vi "Remove Unnecessary Whitespace from XML.vi"(1 "Input":string) -> (0 "Output":string)   [LabVIEW 2018, in "VILab.lvlib"]
doc: "For easier comparison with generated XML to diagnose issues."
uses:
  VILab.lvlib
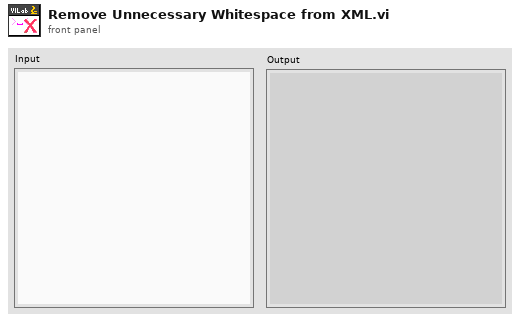
[diagram p1: front panel]
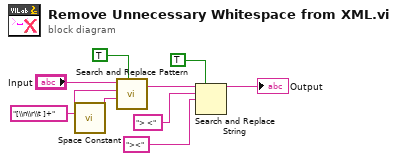
[diagram p0: block diagram]
diagram:
  n1 = call <vilib>:"Space Constant.vi"() -> ("String"=w1:string)
  n2 = call <vilib>:"Search and Replace Pattern.vi"("string"="Input", "regular expression (\"\")"="[\\n\\r\\t ]+", "replace string (\"\")"=w1, "replace all? (F)"=TRUE) -> ("result string"=w6:string)  [unwired: 1 in, 1 out]
  n3 = Search and Replace String(replace all?=TRUE ("replace all? (F)"), input string=w6, search string="> <", replace string="><") -> (result string=→"Output":string)  [unwired: 4 in, 3 out]
